vi "Delete DVR.vi"(8 "Error in":errorcluster, 11 "DVR In":refnum<data-value>) -> (0 "error out":errorcluster)   [LabVIEW 2020, in "Test.lvclass"]
uses:
  Test.lvclass
panel:
  out "Test out":refnum<class "Test.lvclass">
  in  "Test in":refnum<class "Test.lvclass">
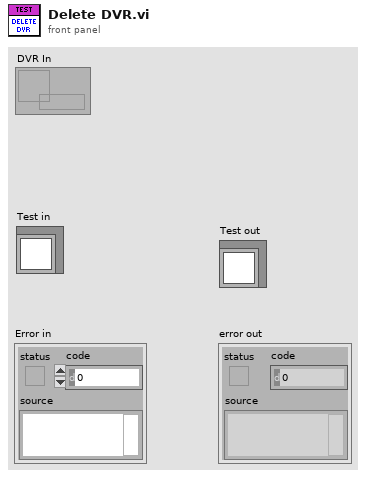
[diagram p1: front panel]
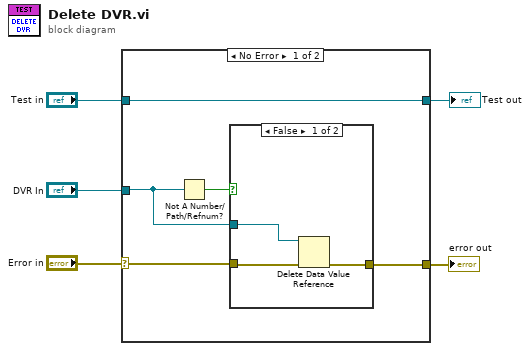
[diagram p0: block diagram]
diagram:
  n1 = case shown="No Error" "Error in" {
    selector: "Error in" -> [w7 w16]
    tunnel: [w6 w16] -> w4
    tunnel: [w10 w15] -> w2
    tunnel: "Test in" -> [w10 w15]
    tunnel: "DVR In" -> [w8 _]
    frame No Error {
      n2 = Not A Number/Path/Refnum?(number/path/refnum=w8) -> (NaN/Path/Refnum?=w9:bool)
      n3 = case shown="False" w9 {
        tunnel: w8 -> [w12 _]
        tunnel: w7 -> [w13 w14]
        tunnel: [w11 w14] -> w6
        frame False {
          n4 = Delete Data Value Reference(data value reference=w12, error in=w13) -> (error out=w11:errorcluster)  [unwired: 1 out]
        }
        frame True {
        }
      }
    }
    frame Error {
    }
  }
  "error out" <- w4
  "Test out" <- w2
